vi "Zapis_ustawien_DI.vi"(8 "error in (no error)":errorcluster, 10 "Kana³y cyfrowe":refnum<vi>, 11 "Plik konf in":path=path "D:/Marek/Dysk Google/Projekty LabVIEW/! Rudpol/Program/Konfiguracja/AI_Konfiguracja.txt") -> (0 "error out":errorcluster, 3 "Plik konf out":path)   [LabVIEW 2014]
doc: "Zapisuje ustawienia kanalow cyfrowych do pliku\nDI_Konfiguracja.txt"
uses:
  Kontrolki/GUI/DI_aktywacja.ctl
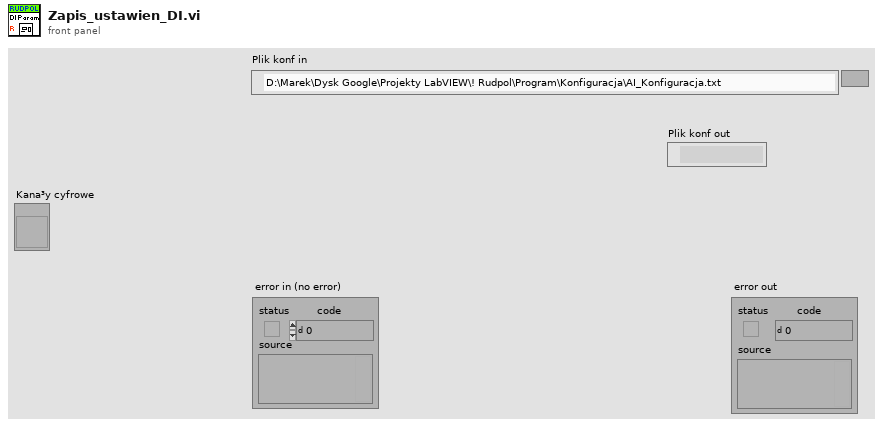
[diagram p1: front panel]
types:
  T1 = enum16{"open", "replace", "create", "open or create", "replace or create", "replace or create with confirmation"}
  T2 = typedef "DI_aktywacja.ctl" = cluster{"DI1":bool, "DI2":bool, "DI3":bool, "DI4":bool, "DI1 Opis":string, "DI2 Opis":string, "DI3 Opis":string, "DI4 Opis":string, "DI1 Amplituda":dbl, "DI2 Amplituda":dbl, "DI3 Amplituda":dbl, "DI4 Amplituda":dbl}
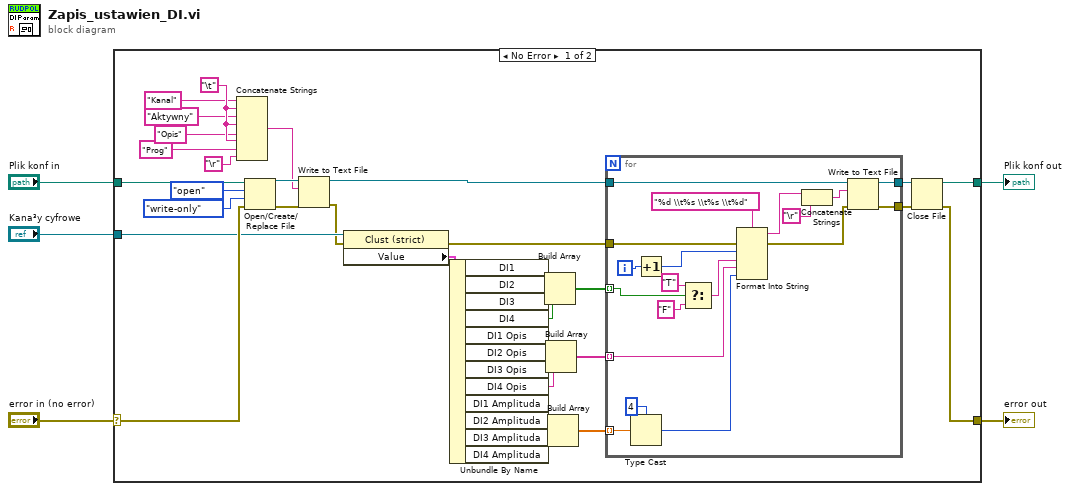
[diagram p0: block diagram]
diagram:
  n1 = case shown="No Error" "error in (no error)" {
    selector: "error in (no error)" -> [w37 w63]
    tunnel: [w6 w63] -> w4
    tunnel: "Kana³y cyfrowe" -> [w28 _]
    tunnel: "Plik konf in" -> [w38 w62]
    tunnel: [w29 w62] -> w2
    frame No Error {
      w36 = "\t"
      n2 = Concatenate Strings("Kanal" ("string"), w36, "Aktywny" ("string"), w36, "Opis" ("string"), w36, "Prog" ("string"), "\r") -> (w30:string)
      n3 = Open/Create/Replace File(file path (use dialog)=w38, error in=w37, operation (0:open)=T1."open", access (0:read/write)=enum16{"read/write", "read-only", "write-only"}."write-only") -> (refnum out=w41:refnum<file>, error out=w42:errorcluster)  [unwired: 2 in, 1 out]
      n4 = Write to Text File(file (use dialog)=w41, text=w30, error in=w42) -> (refnum out=w10:refnum<file>, error out=w27:errorcluster)  [unwired: 1 in, 1 out]
      n5 = property class="Clust (strict)"(reference=w28, error in=w27) -> (error out=w9:errorcluster, "Value"=w26:T2)  [unwired: 1 out]
      n6 = Unbundle By Name(w26) -> ("DI1"=w25:bool, "DI2"=w24:bool, "DI3"=w23:bool, "DI4"=w22:bool, "DI1 Opis"=w21:string, "DI2 Opis"=w20:string, "DI3 Opis"=w19:string, "DI4 Opis"=w18:string, "DI1 Amplituda"=w17:dbl, "DI2 Amplituda"=w16:dbl, "DI3 Amplituda"=w15:dbl, "DI4 Amplituda"=w14:dbl)
      n7 = Build Array(w25, w24, w23, w22) -> (w11:bool[])
      n8 = Build Array(w21, w20, w19, w18) -> (w12:string[])
      n9 = Build Array(w17, w16, w15, w14) -> (w13:dbl[])
      n10 = for {
        tunnel: w13 -> [w45] mode=indexing
        tunnel: w12 -> [w53] mode=indexing
        tunnel: w11 -> [w56] mode=indexing
        tunnel: w10 -> [w50]
        tunnel: w9 -> [w60]
        tunnel: [w51] -> w8
        tunnel: [w49] -> w7
        i -> [w61]
        n11 = Type Cast(type=u8 4 ("upper limit"), x=w45) -> (*(type *) &x=w43:u8)
        n12 = Increment(x=w61) -> (x+1=w58:i32)
        n13 = Select(t="T" ("string"), s=w56, f="F" ("string")) -> (s? t:f=w54:string)
        n14 = Format Into String(format string="%d \\t%s \\t%s \\t%d", error in=w60, w58, w54, w53, w43) -> (resulting string=w46:string, error out=w47:errorcluster)  [unwired: 1 in]
        n15 = Concatenate Strings(w46, "\r") -> (w48:string)
        n16 = Write to Text File(file (use dialog)=w50, text=w48, error in=w47) -> (refnum out=w49:refnum<file>, error out=w51:errorcluster)  [unwired: 1 in, 1 out]
      }
      n17 = Close File(refnum=w7, error in=w8) -> (path=w29:path, error out=w6:errorcluster)
    }
    frame Error {
    }
  }
  "error out" <- w4
  "Plik konf out" <- w2
